vi "Stop.vi"(8 "error in (no error)":errorcluster, 9 "event in":variant, 10 "timeout ms":i32, 11 "VI in":refnum<vi>) -> (0 "error out":errorcluster)   [LabVIEW 2019, in "TemplateModule.lvlib"]
uses:
  TemplateModule.lvlib
  Tools/Tools.lvlib
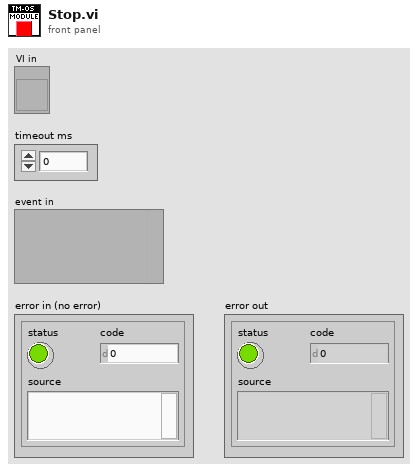
[diagram p1: front panel]
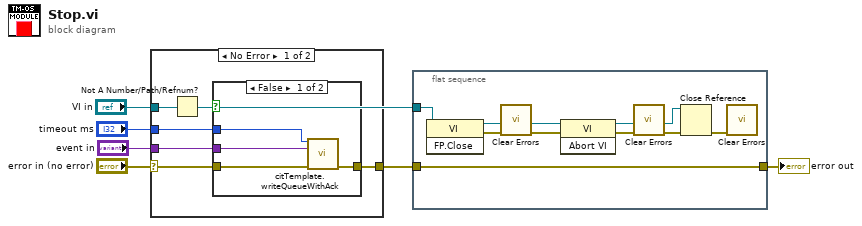
[diagram p0: block diagram]
diagram:
  n1 = case shown="No Error" "error in (no error)" {
    selector: "error in (no error)" -> [w12 w18]
    tunnel: [w10 w18] -> w2
    tunnel: "VI in" -> [w11 _]
    tunnel: "timeout ms" -> [w8 _]
    tunnel: "event in" -> [w7 _]
    frame No Error {
      n2 = Not A Number/Path/Refnum?(number/path/refnum=w11) -> (NaN/Path/Refnum?=w9:bool)
      n3 = case shown="False" w9 {
        tunnel: w12 -> [w16 w17]
        tunnel: [w15 w17] -> w10
        tunnel: w8 -> [w14 _]
        tunnel: w7 -> [w13 _]
        frame False {
          n4 = call "citTemplate.writeQueueWithAck.vi"("timeout ms (-1)"=w14, "event in"=w13, "error in (no error)"=w16) -> ("error out"=w15:errorcluster)  [unwired: 10 in, 2 out]
        }
        frame True {
        }
      }
    }
    frame Error {
    }
  }
  n5 = flat-sequence {
    tunnel: w2 -> [w27]
    tunnel: "VI in" -> [w21]
    tunnel: [w27] -> w3
    frame #0 {
      n6 = invoke class="VI" method="FP.Close"(reference=w21) -> (reference out=w25:refnum<vi>, error out=w26:errorcluster)  [unwired: 2 in, 1 out]
      n7 = call <vilib>:"Clear Errors.vi"("error in (no error)"=w26) -> ("error out"=w24:errorcluster)  [unwired: 5 in, 1 out]
      n8 = invoke class="VI" method="Abort VI"(reference=w25, error in=w24) -> (reference out=w20:refnum<vi>, error out=w23:errorcluster)  [unwired: 1 in, 1 out]
      n9 = call <vilib>:"Clear Errors.vi"("error in (no error)"=w23) -> ("error out"=w22:errorcluster)  [unwired: 5 in, 1 out]
      n10 = Close Reference(reference=w20, error in (no error)=w22) -> (error out=w19:errorcluster)
      n11 = call <vilib>:"Clear Errors.vi"("error in (no error)"=w19) -> ()  [unwired: 5 in, 2 out]
    }
  }
  "error out" <- w3
